vi "current_position.vi"() -> ()   [LabVIEW 2013]
panel:
  in  "y":dbl format="%#_13g"
  in  "x":dbl format="%#_13g"
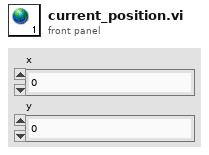
[diagram p1: front panel]
diagram:
